vi "Entry.vi"(8 "error in (no error)":errorcluster, 11 "New State":refnum<class "Starting Command.lvclass">) -> (0 "error out":errorcluster, 3 "State out":refnum<class "Starting Command.lvclass">)   [LabVIEW 2014, in "Robot Actor Framework.lvlib" / "Command Processor Actor.lvlib" / "Starting Command.lvclass"]
doc: "This is an abstract method. Override this method to define the behavior when you enter the state."
uses:
  Starting Command.lvclass
  Command Processor Actor Class/Command Processor States.ctl
  <vilib>/ActorFramework/Actor/Actor.lvclass/Actor.ctl
  System Actor/System Actor Messages/Write Current Command Msg/Write Current Command Msg.lvclass/Write Current Command Msg.ctl
  <vilib>/ActorFramework/Message Enqueuer/Message Enqueuer.lvclass/Message Enqueuer.ctl
  <vilib>/ActorFramework/Message Enqueuer/Enqueue.vi
  <vilib>/ActorFramework/Message Priority Queue/Priority Enqueue.vi
  System Actor/System Actor Messages/Write Current Command Msg/Write Current Command Msg.lvclass
  Command Processor Actor Class/Command Processor Actor.lvclass
  <vilib>/ActorFramework/Actor/Actor.lvclass
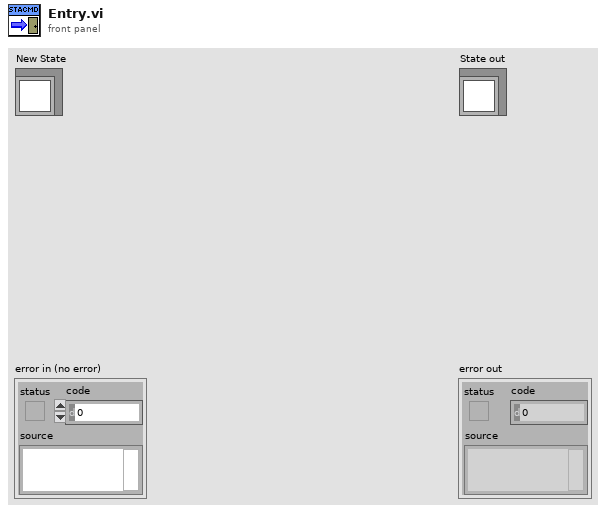
[diagram p1: front panel]
types:
  T1 = typedef "Robot Actor Framework.lvlib/Command Processor Actor.lvlib/Command Processor Actor.lvclass/Command Processor States.ctl" = enum16{"Unknown", "No Command", "Running Command", "Starting Command", "Stopping Command", "Finishing Command"}
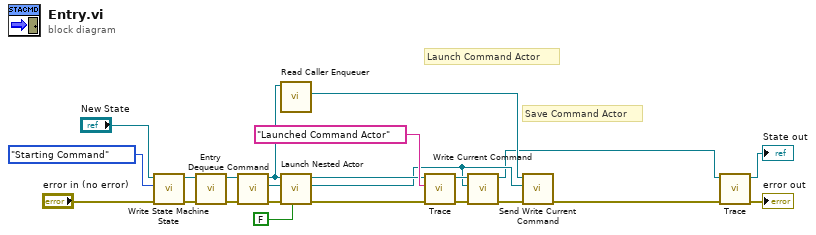
[diagram p0: block diagram]
diagram:
  # "Save Command Actor"
  # "Launch Command Actor"
  n1 = call-dynamic "Write State Machine State.vi"("error in (no error)"="error in (no error)", "Command Processor State"=Command_Processor_States."Starting Command", "Command Processor Actor in"="New State") -> ("error out"=w18:errorcluster, "Command Processor Actor out"=w19:refnum<class "Starting Command.lvclass">)  [unwired: 7 in]
  n2 = call-parent "Entry.vi"("error in (no error)"=w18, "New State"=w19) -> ("error out"=w16:errorcluster, "State out"=w17:refnum<class "Starting Command.lvclass">)  [unwired: 8 in]
  n3 = call-dynamic "Dequeue Command.vi"("error in (no error)"=w16, "Command Processor Actor in"=w17) -> ("error out"=w1:errorcluster, "Command"=w2:refnum<class "Command Actor.lvclass">, "Command Processor Actor out"=w9:refnum<class "Starting Command.lvclass">)  [unwired: 7 in]
  n4 = call <vilib>:"Read Caller Enqueuer.vi"("Actor"=w9) -> ("Caller Enqueuer"=w8:refnum<class "Message Enqueuer.lvclass">)  [unwired: 10 in]
  n5 = call <vilib>:"Launch Nested Actor.vi"("Open Actor Core front panel? (F)"=FALSE, "error in (no error)"=w1, "Nested Actor"=w2, "Caller Actor in"=w9) -> ("error out"=w12:errorcluster, "Nested Actor's Enqueuer"=w7:refnum<class "Message Enqueuer.lvclass">, "Caller Actor out"=w10:refnum<class "Starting Command.lvclass">)  [unwired: 5 in]
  n6 = call-dynamic "Trace.vi"("error in (no error)"=w12, "Command Processor Action"="Launched Command Actor", "Command Processor Actor in"=w10) -> ("error out"=w11:errorcluster, "Command Processor Actor out"=w15:refnum<class "Starting Command.lvclass">)  [unwired: 7 in]
  n7 = call-dynamic "Write Current Command.vi"("error in (no error)"=w11, "Actor Framework:Message Enqueuer"=w7, "Command Processor in"=w15) -> ("error out"=w13:errorcluster, "Command Processor out"=w4:refnum<class "Starting Command.lvclass">)  [unwired: 7 in]
  n8 = call "Send Write Current Command.vi"("error in (no error)"=w13, "Actor Framework:Message Enqueuer"=w7, "Message Enqueuer"=w8) -> ("error out"=w6:errorcluster)  [unwired: 7 in, 1 out]
  n9 = call-dynamic "Trace.vi"("error in (no error)"=w6, "Command Processor Actor in"=w4) -> ("error out"=→"error out":errorcluster, "Command Processor Actor out"=→"State out":refnum<class "Starting Command.lvclass">)  [unwired: 8 in]
